vi "HK Channel Read CVT Settings.vi"(8 "error in (no error)":errorcluster, 11 "HK Channel in":refnum<class "HK Table.lvclass">) -> (0 "error out":errorcluster, 2 "CVT Settings":T1 {"Max Age" format="%<%H:%M:%S>t"}, 3 "HK Channel out":refnum<class "HK Table.lvclass">)   [LabVIEW 2019, in "HK Table.lvclass"]
uses:
  HK Table.lvclass
  HK Current Value Table Settings.ctl
  HK Table.lvclass/HK Table.ctl
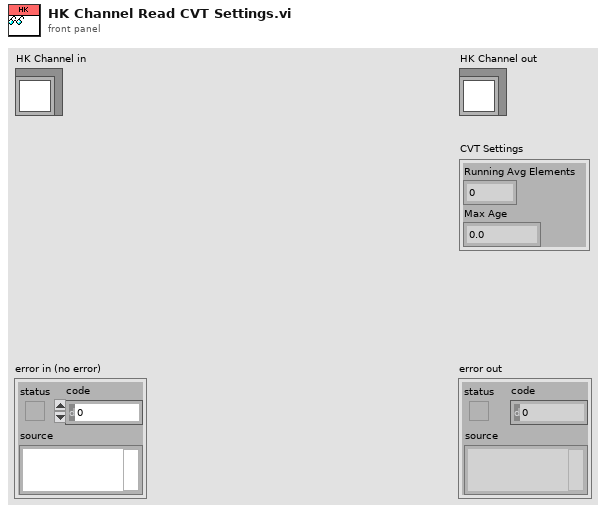
[diagram p1: front panel]
types:
  T1 = typedef "HK Table.lvclass/HK Current Value Table Settings.ctl" = cluster{"Running Avg Elements":i32, "Max Age":dbl}
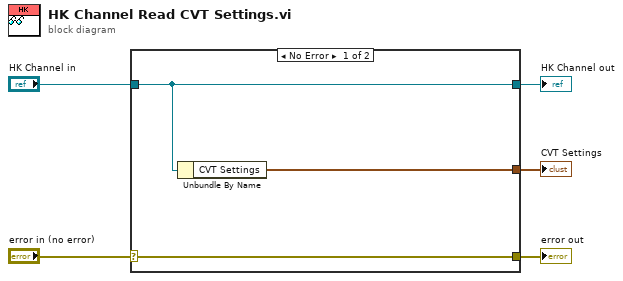
[diagram p0: block diagram]
diagram:
  n1 = case shown="No Error" "error in (no error)" {
    selector: "error in (no error)" -> [w8 w9]
    tunnel: [w8 w9] -> w4
    tunnel: [w7 w10] -> w2
    tunnel: "HK Channel in" -> [w7 w10]
    tunnel: [w6 _] -> w1
    frame No Error {
      n2 = Unbundle By Name(w7) -> ("CVT Settings"=w6:T1)
    }
    frame Error {
    }
  }
  "error out" <- w4
  "HK Channel out" <- w2
  "CVT Settings" <- w1
